vi "Solution.vi"() -> ()   [LabVIEW 2020]
panel:
  in  "part 2?":bool
  out "progress":dbl
  in  "input":string
  out "result":u64
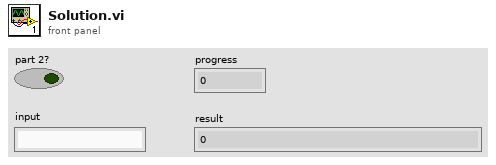
[diagram p1: front panel]
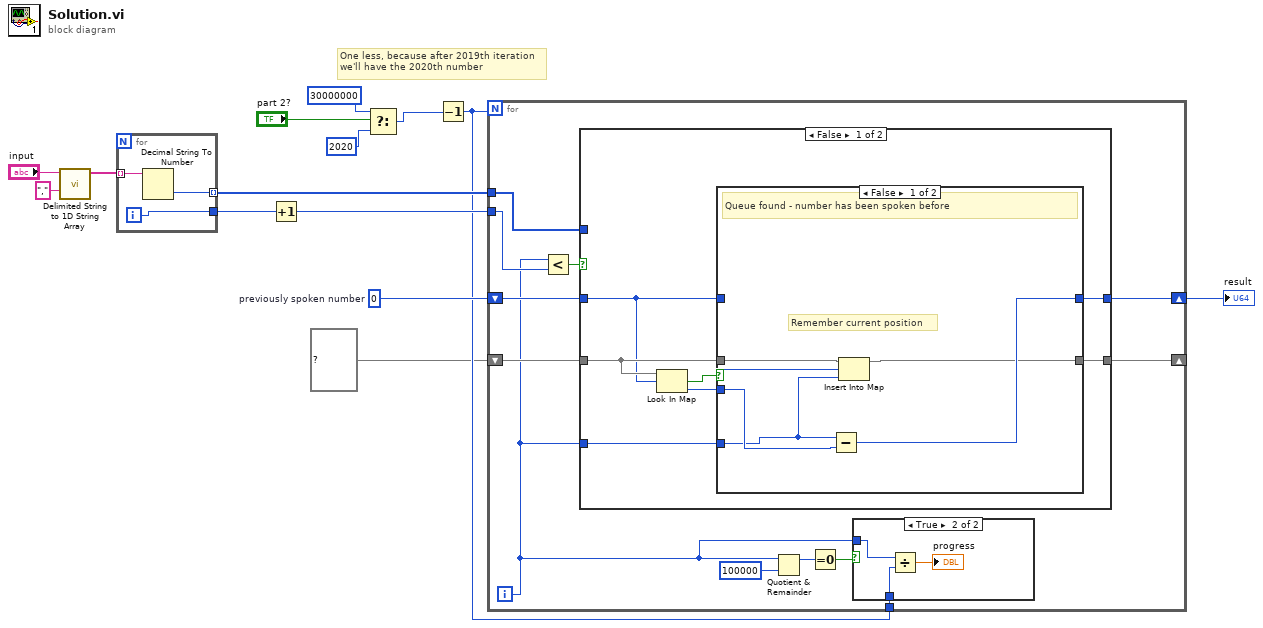
[diagram p0: block diagram]
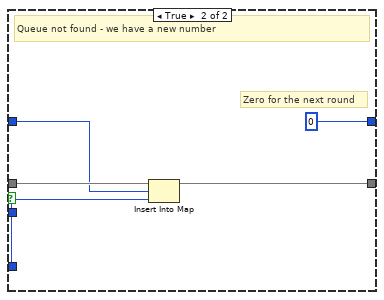
[diagram p2: hidden frame]
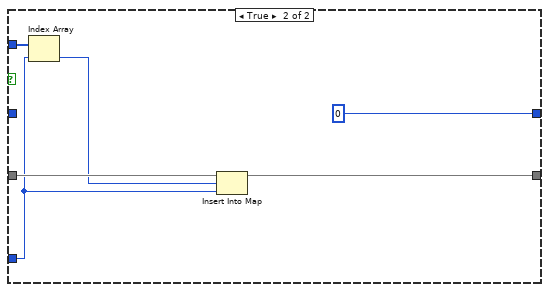
[diagram p3: hidden frame]
diagram:
  w7 = 0  # previously spoken number
  # "One less, because after 2019th iteration\nwe'll have the 2020th number"
  n1 = call <vilib>:"Delimited String to 1D String Array.vi"("delimiter"=",", "delimited string"="input") -> ("string array"=w12:string[])  [unwired: 9 in]
  n2 = for {
    tunnel: w12 -> [w17] mode=indexing
    tunnel: [w16] -> w11 mode=indexing
    tunnel: [w15] -> w9
    i -> [w15]
    n3 = Decimal String To Number(string=w17) -> (number=w16:i32)  [unwired: 2 in, 1 out]
  }
  n4 = Increment(x=w9) -> (x+1=w10:i32)
  n5 = Select(t=30000000, s="part 2?", f=2020) -> (s? t:f=w3:i32)
  n6 = Decrement(x=w3) -> (x-1=w5:i32)
  n7 = for {
    N: w5 -> [_]
    tunnel: w11 -> [w29]
    tunnel: w10 -> [w28]
    shift-right: [w23] -> w6
    shift-left: w7 -> [w24]
    shift-right: [w25] -> _
    shift-left: map{u64, u64} {} ("memory") -> [w26]
    tunnel: w5 -> [w18]
    i -> [w19]
    n8 = Less?(x=w19, y=w28) -> (x < y?=w27:bool)
    n9 = case shown="False" w27 {
      tunnel: w29 -> [_ w53]
      tunnel: w19 -> [w34 w48]
      tunnel: [w30 0] -> w23
      tunnel: w26 -> [w35 w52]
      tunnel: [w33 w50] -> w25
      tunnel: w24 -> [w32 _]
      frame False {
        n10 = Look In Map(map=w35, key=w32) -> (key not found?=w36:bool, value=w31:u64)  [unwired: 1 in]
        n11 = case shown="False" w36 {
          tunnel: w35 -> [w41 w47]
          tunnel: w34 -> [w38 w43]
          tunnel: [w40 w46] -> w33
          tunnel: w32 -> [w37 w45]
          tunnel: w31 -> [w39 _]
          tunnel: [w42 0] -> w30
          frame False {
            # "Remember current position"
            # "Queue found - number has been spoken before"
            n12 = Subtract(x=w38, y=w39) -> (x-y=w42:u64)
            n13 = Insert Into Map(map in=w41, key=w37, value=w38) -> (map out=w40:map{u64, u64})  [unwired: 2 out]
          }
          frame True {
            # "Zero for the next round"
            # "Queue not found - we have a new number"
            n14 = Insert Into Map(map in=w47, key=w45, value=w43) -> (map out=w46:map{u64, u64})  [unwired: 2 out]
          }
        }
      }
      frame True {
        n15 = Index Array(array=w53, index=w48) -> (element=w51:i32)
        n16 = Insert Into Map(map in=w52, key=w51, value=w48) -> (map out=w50:map{u64, u64})  [unwired: 2 out]
      }
    }
    n17 = Quotient & Remainder(x=w19, y=100000) -> (x-y*floor(x/y)=w20:i32)  [unwired: 1 out]
    n18 = Equal To 0?(x=w20) -> (x = 0?=w21:bool)
    n19 = case shown="True" w21 {
      tunnel: w19 -> [_ w56]
      tunnel: w18 -> [_ w55]
      frame False {
      }
      frame True {
        n20 = Divide(x=w56, y=w55) -> (x/y=→"progress":dbl)
      }
    }
  }
  "result" <- w6
